vi "test_Particle Filter_calib.vi"() -> (2 "Array":T1(array[cluster]))   [LabVIEW 2020]
doc: "This example performs a series of grayscale filtering, threshold, binary morphology, and particle analysis operations to measure the areas of all the large circular particles of the image."
uses:
  <vilib>/vision/NI_Vision_Development_Module.lvlib
panel:
  in  "Range":cluster{"Lower value":sgl, "Upper value":sgl}={"Lower value"=40.0, "Upper value"=255.0}
  in  "Tab Control":T2(tab)
  out "Original":T3(plugin-control) caption="Original Image"
  out "Threshold":T3(plugin-control) caption="Threshold Image"
  out "Fill Hole and Reject Border":T3(plugin-control) caption="Reject Border and Fill Holes"
  out "Filter and Overlay Area":T3(plugin-control) caption="Filter Out Non Circles and Overlay Particle Area"
  # "Overview: Demonstrates how to use the IMAQ Particle Filter and other functions to remove unwanted particles from a binary image, and then IMAQ Particle Analysis is used to calculate the location and area of the remaining particles to overlay the results on the image. \nRequirements: Vision Development Software.\nInstructions: Run the VI, and click on the different tabs to see how the image is processed."
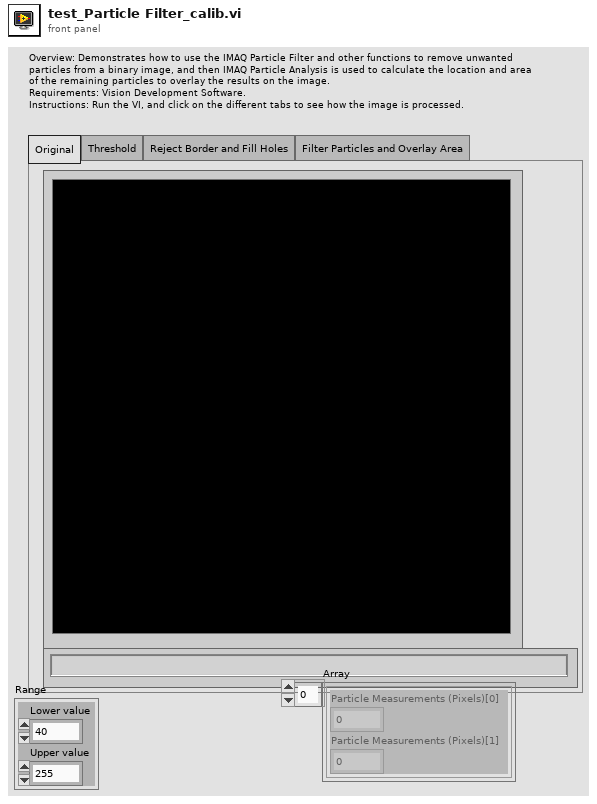
[diagram p1: front panel]
types:
  T1 = cluster{"Particle Measurements (Pixels)[0]":dbl, "Particle Measurements (Pixels)[1]":dbl}[]
  T2 = enum32{"Original", "Threshold", "Reject Border and Fill Holes", "Filter Particles and Overlay Area"}
  T3 = typedef "IMAQ Image.ctl" = refnum<image>
  T4 = typedef "Particle Parameters" = i32
  T5 = cluster{"Measurement Parameter":T4, "Range Lower Value":dbl, "Range Upper Value":dbl, "Range":bool, "Measurement Type":bool}[]
  T6 = cluster{"Desired Font (Application)":enum16{"User-specified Font", "Application Font", "System Font", "Dialog Font"}, "[User-specified Font]":cluster{"Font Name":string, "Size":i16, "Strikeout?":bool, "Italic?":bool, "Underline?":bool, "Outline?":bool, "Shadow?":bool, "Bold?":bool, "Rotation Angle":dbl}, "Horizontal Alignment":i16, "Vertical Alignment":i16}
  T7 = cluster{"Particle Measurements (Pixels)[0]":dbl, "Particle Measurements (Pixels)[1]":dbl, "Particle Measurements (Pixels)[2]":dbl}
  T8 = cluster{"Particle Measurements (Pixels)[0]":dbl, "Particle Measurements (Pixels)[1]":dbl}
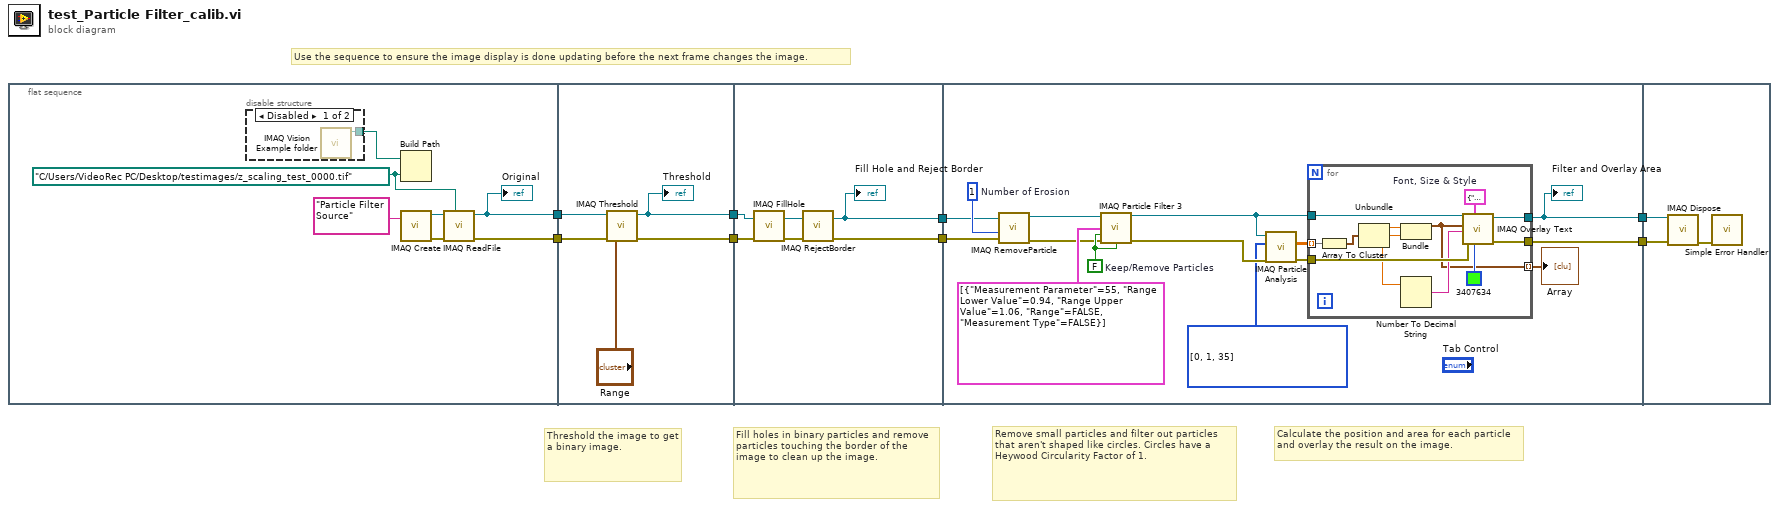
[diagram p0: block diagram]
diagram:
  # "Use the sequence to ensure the image display is done updating before the next frame changes the image."
  # "Calculate the position and area for each particle and overlay the result on the image."
  # "Remove small particles and filter out particles that aren't shaped like circles. Circles have a Heywood Circularity Factor of 1."
  # "Fill holes in binary particles and remove particles touching the border of the image to clean up the image."
  # "Threshold the image to get a binary image."
  n1 = flat-sequence {
    tunnel: [w11] -> w4
    tunnel: [w10] -> w3
    tunnel: [w20] -> w8
    tunnel: [w21] -> w7
    tunnel: w4 -> [w19]
    tunnel: w3 -> [w18]
    tunnel: w8 -> [w27]
    tunnel: w7 -> [w26]
    tunnel: [w22] -> w6
    tunnel: [w23] -> w5
    tunnel: w5 -> [w31]
    tunnel: w6 -> [w30]
    tunnel: [w37] -> w2
    tunnel: [w29] -> w1
    tunnel: w2 -> [w56]
    tunnel: w1 -> [w57]
    frame #0 {
      w9 = path "C:/Users/VideoRec PC/Desktop/testimages/z_scaling_test_0000.tif" ("name or relative path")
      n2 = disable-structure shown="Disabled" {
        disable-tunnel: [w16 _] -> w15
        frame Disabled {
          n3 = call "IMAQ Vision Example folder.vi"() -> ("Example Image Path"=w16:path)  [unwired: 11 in]
        }
        frame Enabled {
        }
      }
      n4 = Build Path(base path=w15, name or relative path=w9) -> ()  [unwired: 1 out]
      n5 = call "IMAQ Create"("Image Name"="Particle Filter Source") -> ("New Image"=w13:T3, "error out"=w12:errorcluster)  [unwired: 4 in]
      n6 = call "IMAQ ReadFile"("File Path"=w9, "error in (no error)"=w12, "Image"=w13) -> ("error out"=w10:errorcluster, "Image Out"=w11:T3)  [unwired: 4 in, 3 out]
      "Original" <- w11
    }
    frame #1 {
      n7 = call "IMAQ Threshold"("error in (no error)"=w18, "Range"="Range", "Image Src"=w19) -> ("error out"=w21:errorcluster, "Image Dst Out"=w20:T3)  [unwired: 7 in]
      "Threshold" <- w20
    }
    frame #2 {
      n8 = call "IMAQ FillHole"("error in (no error)"=w26, "Image Src"=w27) -> ("error out"=w24:errorcluster, "Image Dst Out"=w25:T3)  [unwired: 4 in]
      n9 = call "IMAQ RejectBorder"("error in (no error)"=w24, "Image Src"=w25) -> ("error out"=w23:errorcluster, "Image Dst Out"=w22:T3)  [unwired: 4 in]
      "Fill Hole and Reject Border" <- w22
    }
    frame #3 {
      w34 = 1  # Number of Erosion
      w36 = FALSE  # Keep/Remove Particles
      w38 = T4[] [0, 1, 35] items=["Center of Mass X", "Center of Mass Y", "First Pixel X", "First Pixel Y", "Bounding Rect Left", "Bounding Rect Top", "Bounding Rect Right", "Bounding Rect Bottom", "Max Feret Diameter Start X", "Max Feret Diameter Start Y", "Max Feret Diameter End X", "Max Feret Diameter End Y", "Max Horiz. Segment Length Left", "Max Horiz. Segment Length Right", "Max Horiz. Segment Length Row", "-", "Bounding Rect Width", "Bounding Rect Height", "Bounding Rect Diagonal", "Perimeter", "Convex Hull Perimeter", "Holes' Perimeter", "Max Feret Diameter", "Equivalent Ellipse Major Axis", "Equivalent Ellipse Minor Axis", "Equivalent Ellipse Minor Axis (Feret)", "Equivalent Rect Long Side", "Equivalent Rect Short Side", "Equivalent Rect Diagonal", "Equivalent Rect Short Side (Feret)", "Average Horiz. Segment Length", "Average Vert. Segment Length", "Hydraulic Radius", "Waddel Disk Diameter", "-", "Area", "Holes' Area", "Particle & Holes' Area", "Convex Hull Area", "Image Area", "-", "Number of Holes", "Number of Horiz. Segments", "Number of Vert. Segments", "-", "Orientation", "Max Feret Diameter Orientation", "-", "% Area/Image Area", "% Area/(Particle & Holes' Area)", "Ratio of Equivalent Ellipse Axes", "Ratio of Equivalent Rect Sides", "-", "Elongation Factor", "Compactness Factor", "Heywood Circularity Factor", "Type Factor", "-", "Sum X", "Sum Y", "Sum XX", "Sum XY", "Sum YY", "Sum XXX", "Sum XXY", "Sum XYY", "Sum YYY", "-", "Moment of Inertia XX", "Moment of Inertia XY", "Moment of Inertia YY", "Moment of Inertia XXX", "Moment of Inertia XXY", "Moment of Inertia XYY", "Moment of Inertia YYY", "Norm. Moment of Inertia XX", "Norm. Moment of Inertia XY", "Norm. Moment of Inertia YY", "Norm. Moment of Inertia XXX", "Norm. Moment of Inertia XXY", "Norm. Moment of Inertia XYY", "Norm. Moment of Inertia YYY", "Hu Moment 1", "Hu Moment 2", "Hu Moment 3", "Hu Moment 4", "Hu Moment 5", "Hu Moment 6", "Hu Moment 7"] ("Pixel Measurements")
      n10 = call "IMAQ RemoveParticle"("error in (no error)"=w31, "Number of Erosion"=w34, "Image Src"=w30) -> ("error out"=w32:errorcluster, "Image Dst Out"=w33:T3)  [unwired: 7 in]
      n11 = call "IMAQ Particle Filter 3"("Image Src"=w33, "Selection Values"=T5 [{"Measurement Parameter"=55, "Range Lower Value"=0.94, "Range Upper Value"=1.06, "Range"=FALSE, "Measurement Type"=FALSE}], "Keep/Remove Particles (F)"=w36, "error in (no error)"=w32, "Fill Holes? (F)"=w36) -> ("Image Dst Out"=w41:T3, "error out"=w42:errorcluster)  [unwired: 8 in, 1 out]
      n12 = call "IMAQ Particle Analysis"("error in (no error)"=w42, "Pixel Measurements"=w38, "Image"=w41) -> ("error out"=w39:errorcluster, "Particle Measurements (Pixels)"=w40:dbl[][])  [unwired: 3 in, 4 out]
      n13 = for {
        tunnel: w39 -> [w55]
        tunnel: [w54] -> w37
        tunnel: [w53] -> w29
        tunnel: w41 -> [w50]
        tunnel: w40 -> [w45] mode=indexing
        tunnel: [w43] -> w28 mode=indexing
        w44 = T6 {"Desired Font (Application)"=enum."Application Font", "[User-specified Font]"={"Font Name"="", "Size"=12, "Strikeout?"=FALSE, "Italic?"=FALSE, "Underline?"=FALSE, "Outline?"=FALSE, "Shadow?"=FALSE, "Bold?"=FALSE, "Rotation Angle"=0.0}, "Horizontal Alignment"=0, "Vertical Alignment"=0}  # Font, Size & Style
        n14 = Array To Cluster(array=w45) -> (cluster=w49:T7)
        n15 = Unbundle(w49) -> ("Particle Measurements (Pixels)[0]"=w48:dbl, "Particle Measurements (Pixels)[1]"=w47:dbl, "Particle Measurements (Pixels)[2]"=w46:dbl)
        n16 = Bundle("Particle Measurements (Pixels)[0]"=w48, "Particle Measurements (Pixels)[1]"=w47) -> (w43:T8)  [unwired: 1 in]
        n17 = Number To Decimal String(number=w46) -> (decimal integer string=w52:string)  [unwired: 1 in]
        n18 = call "IMAQ Overlay Text"("Text Color (black)"=u32 3407634, "Font, Size & Style"=w44, "error in (no error)"=w55, "String"=w52, "Origin"=w43, "Image"=w50) -> ("error out"=w54:errorcluster, "Image Out"=w53:T3)  [unwired: 4 in]
      }
      "Filter and Overlay Area" <- w29
      "Array" <- w28
    }
    frame #4 {
      n19 = call "IMAQ Dispose"("Image"=w57, "error in (no error)"=w56) -> ("error out"=w58:errorcluster)  [unwired: 4 in]
      n20 = call <vilib>:"Simple Error Handler.vi"("error in (no error)"=w58) -> ()  [unwired: 4 in, 5 out]
    }
  }
